vi "Check Sample Transfer Controls.vi"(6 "Push Source Storage":T1, 7 "Sample Push State":T2=enum."Idle", 8 "error in (no error)":errorcluster, 9 "Target Container":T1, 10 "Source Container":T1, 11 "cRIO-CO2 in":refnum<class "cRIO-CO2.lvclass">) -> (0 "error out":errorcluster, 1 "Target Container":T1=enum."Undefined", 2 "Source Container":T1=enum."Undefined", 3 "cRIO-CO2 out":refnum<class "cRIO-CO2.lvclass">, 5 "Containers check":T3)   [LabVIEW 2015, in "cRIO-Carbondioxide.lvlib" / "cRIO-CO2.lvlib" / "cRIO-CO2.lvclass"]
uses:
  cRIO-CO2.lvclass
  Controls/Sample Transfer Container Enumerator.ctl
  Controls/Containers Check Enumerator.ctl
  Controls/Sample Push State Enumerator.ctl
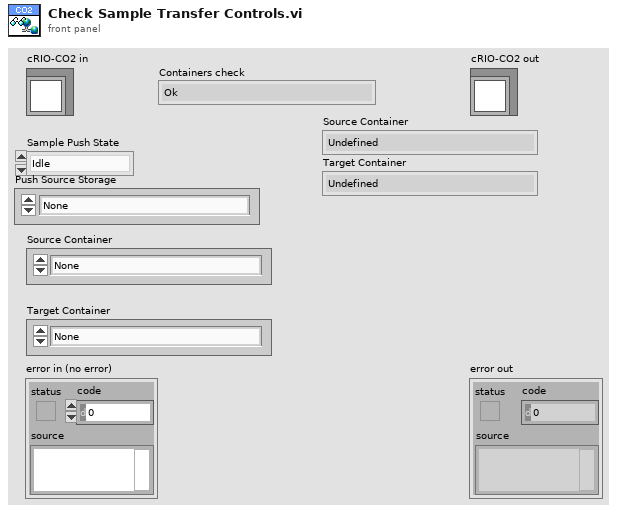
[diagram p1: front panel]
types:
  T1 = typedef "Sample Transfer Container Enumerator.ctl" = enum16{"None", "Sample 1", "Sample 2", "Sample 3", "Sample 4", "Sample 5", "Storage 01", "Storage 02", "Storage 03", "Storage 04", "Storage 05", "Storage 06", "Storage 07", "Storage 08", "Storage 09", "Storage 10", "Storage 11", "Storage 12", "Syringe", "Undefined"}
  T2 = typedef "Sample Push State Enumerator.ctl" = enum16{"Undefined", "Initialize", "Dilute", "Close Transfer Line", "Start Heaters", "Warm Up Syringe", "Ready to Push", "Push", "Initiate Stash", "Stash", "Complete", "Abort", "Idle", "Error"}
  T3 = typedef "Containers Check Enumerator.ctl" = enum16{"Ok", "Same", "Undefined", "Invalid Target", "Invalid Push State", "Invalid Source Sample"}
  T4 = enum16{"Ok", "Same", "Undefined", "Invalid Target"}
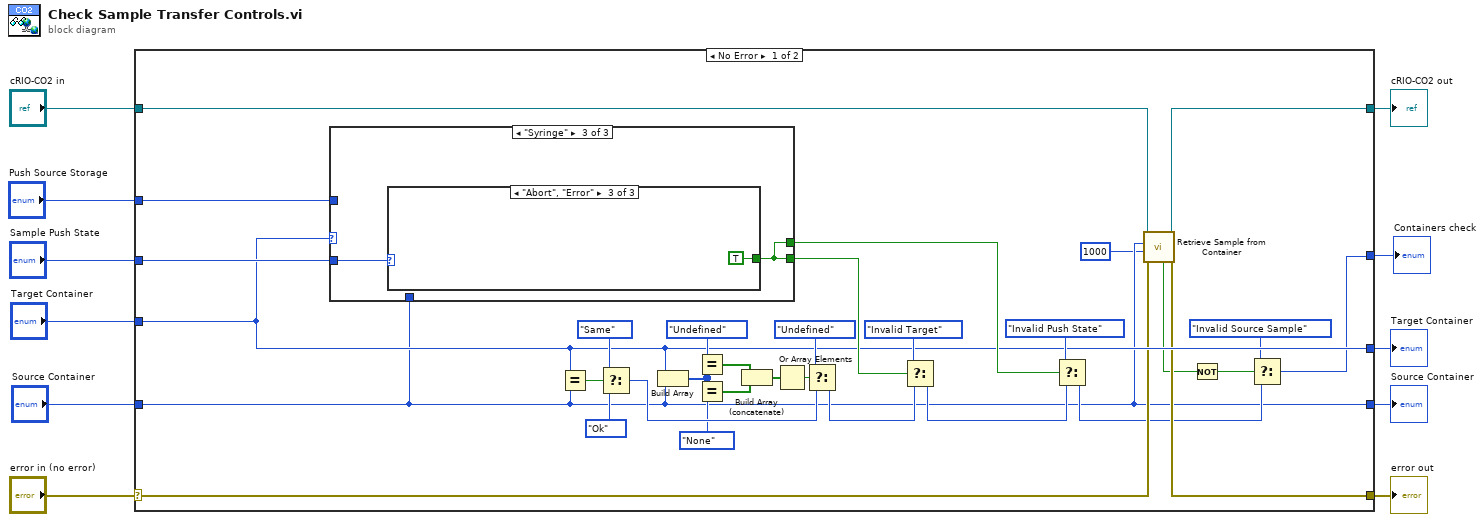
[diagram p0: block diagram]
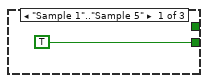
[diagram p2: hidden frame]
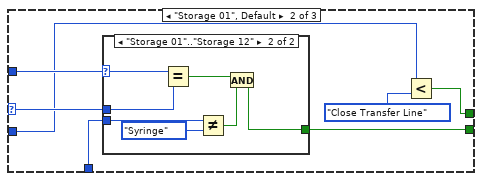
[diagram p3: hidden frame]
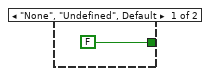
[diagram p4: hidden frame]
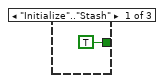
[diagram p5: hidden frame]
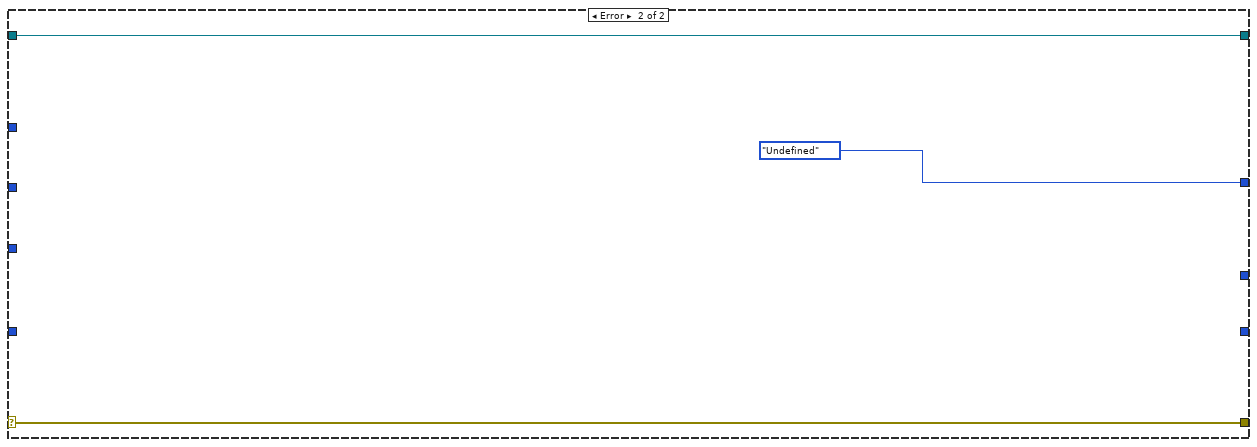
[diagram p7: hidden frame]
diagram:
  n1 = case shown="No Error" "error in (no error)" {
    selector: "error in (no error)" -> [w21 w66]
    tunnel: [w20 w66] -> w10
    tunnel: [w22 w65] -> w8
    tunnel: "cRIO-CO2 in" -> [w23 w65]
    tunnel: [w14 _] -> w7
    tunnel: [w24 _] -> w6
    tunnel: [w17 T4."Undefined" ("f")] -> w5
    tunnel: "Sample Push State" -> [w26 _]
    tunnel: "Target Container" -> [w24 _]
    tunnel: "Source Container" -> [w14 _]
    tunnel: "Push Source Storage" -> [w25 _]
    frame No Error {
      n2 = case shown="\"Syringe\"" w24 {
        selector: w24 -> [_ w50 _]
        tunnel: [TRUE w48 w60] -> w37
        tunnel: w26 -> [_ w46 w61]
        tunnel: [_ w47 w60] -> w29
        tunnel: w25 -> [_ w51 _]
        tunnel: w14 -> [_ w49 _]
        frame "Sample 1".."Sample 5" {
        }
        frame "Storage 01", Default {
          n3 = case shown="\"Storage 01\"..\"Storage 12\"" w51 {
            selector: w51 -> [_ w59]
            tunnel: [FALSE w53] -> w48
            tunnel: w50 -> [_ w58]
            tunnel: w49 -> [_ w56]
            frame "None", "Undefined", Default {
            }
            frame "Storage 01".."Storage 12" {
              n4 = Equal?(x=w59, y=w58) -> (x = y?=w57:bool)
              n5 = Not Equal?(x=w56, y=Sample_Transfer_Container_Enumerator."Syringe") -> (x != y?=w54:bool)
              n6 = And(x=w57, y=w54) -> (x .and. y?=w53:bool)
            }
          }
          n7 = Less?(x=w46, y=Sample_Push_State_Enumerator."Close Transfer Line") -> (x < y?=w47:bool)
        }
        frame "Syringe" {
          n8 = case shown="\"Abort\", \"Error\"" w61 {
            tunnel: [TRUE _ TRUE] -> w60
            frame "Initialize".."Stash" {
            }
            frame "Undefined", "Complete", "Idle" {
            }
            frame "Abort", "Error" {
            }
          }
        }
      }
      n9 = Equal?(x=w24, y=w14) -> (x = y?=w43:bool)
      n10 = Select(t=Containers_Check_Enumerator."Same" ("Containers check"), s=w43, f=Containers_Check_Enumerator."Ok") -> (s? t:f=w36:T3)
      n11 = Build Array(w24, w14) -> (w32:T1[])
      n12 = Equal?(x=Sample_Transfer_Container_Enumerator."Undefined" ("data out"), y=w32) -> (x = y?=w31:bool[])
      n13 = Equal?(x=w32, y=Sample_Transfer_Container_Enumerator."None" ("data out")) -> (x = y?=w30:bool[])
      n14 = Build Array (concatenate)(w31, w30) -> (w33:bool[])
      n15 = Or Array Elements(Boolean array=w33) -> (logical OR=w41:bool)
      n16 = Select(t=Containers_Check_Enumerator."Undefined" ("Containers check"), s=w41, f=w36) -> (s? t:f=w28:T3)
      n17 = Select(t=Containers_Check_Enumerator."Invalid Target", s=w37, f=w28) -> (s? t:f=w18:T3)
      n18 = Select(t=Containers_Check_Enumerator."Invalid Push State", s=w29, f=w18) -> (s? t:f=w15:T3)
      n19 = call "Retrieve Sample from Container.vi"("error in (no error)"=w21, "timeout in ms (1000)"=1000 ("timeout in ms (-1)"), "Sample Container"=w14, "cRIO-CO2 in"=w23) -> ("error out"=w20:errorcluster, "cRIO-CO2 out"=w22:refnum<class "cRIO-CO2.lvclass">, "Valid Sample (Not Empry nor Dirt)"=w16:bool)  [unwired: 3 in, 2 out]
      n20 = Not(x=w16) -> (.not. x?=w13:bool)
      n21 = Select(t=Containers_Check_Enumerator."Invalid Source Sample", s=w13, f=w15) -> (s? t:f=w17:T3)
    }
    frame Error {
    }
  }
  "error out" <- w10
  "cRIO-CO2 out" <- w8
  "Source Container" <- w7
  "Target Container" <- w6
  "Containers check" <- w5
